vi "PH_Tektronix_7000.get Acquisition Configuration.vi"(0 "i ref in":refnum<vi>, 5 "error IO":errorcluster) -> (14 "i ref out":refnum<vi>, 19 "error out":errorcluster)   [LabVIEW 2014, in "PH_Tektronix_7000.lvlib"]
doc: "If the connection is established, the acquisition configuration is queried from the hardware and written to own attributes as well as the errors."
uses:
  PH_Tektronix_7000.lvlib
  PH_Tektronix_7000.Acquisition Config.ctl
  instr.lib/Tektronix7000Series/Tektronix 7000 Series - Driver np.lvlib
panel:
  in  "Acquisition Configuration":T1={"Record Length"=10000, "Timebase [s/div]"=4.0, "Position [%]"=0.0, "Acquisition Type"=0, "Average Waveforms"=10, "Envelope Waveforms"=10, "WfmDB Samples"=16000, "Continuous?"=FALSE, "Delay [s]"=0.0, "Run?"=FALSE} {"Delay [s]" format="%#_12p"; "Acquisition Type" items=["Sample", "Peak Detect", "Hi Res", "Average", "Envelope", "WfmDB"]; "Timebase [s/div]" format="%#_12g"}
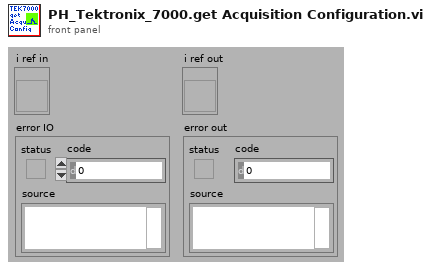
[diagram p1: front panel]
types:
  T1 = typedef "PH_Tektronix_7000.lvlib/PH_Tektronix_7000.Acquisition Config.ctl" = cluster{"Record Length":u32, "Timebase [s/div]":dbl, "Position [%]":dbl, "Acquisition Type":u16, "Average Waveforms":i32, "Envelope Waveforms":i32, "WfmDB Samples":i32, "Continuous?":bool, "Delay [s]":dbl, "Run?":bool}
  T2 = typedef "PH_Tektronix_7000.lvlib/PH_Tektronix_7000.i attribute.ctl" = cluster{"VISA Resource Name":refnum<visa-resource-name>, "IDN":cluster{"Instrument Driver":string, "Instrument Firmware":string, "Model":string, "Serial Number":string}, "Selftest":cluster{"Result":i32, "Message":string}, "Trigger Configuration":T3, "Acquisition Configuration":T1, "GUI Refs":T4, "State":T5, "Error Message":string, "Allow Prdc Loop?":bool, "Channel 1":T6, "Channel 2":T6, "Channel 3":T6, "Channel 4":T6, "Data CH 1":waveform(dbl), "Data CH 2":waveform(dbl), "Data CH 3":waveform(dbl), "Data CH 4":waveform(dbl), "Allow config?":bool, "Name Channel 1":string, "Name Channel 2":string, "Name Channel 3":string, "Name Channel 4":string, "Fetch Data before sending to PSDB?":bool, "Constructor passed?":bool, "Data taken at":timestamp, "Plot Colors":u32[], "Default VISA Resource":string}
  T3 = typedef "PH_Tektronix_7000.lvlib/PH_Tektronix_7000.Trigger Config.ctl" = cluster{"Source":u16, "Level [V]":dbl, "Slope":u16, "Coupling":u16, "Trigger Mode":u16}
  T4 = typedef "PH_Tektronix_7000.lvlib/PH_Tektronix_7000.GUI Refs.ctl" = cluster{"Graph":refnum<vi>, "State":refnum<vi>, "Delete":refnum<vi>, "VISA Resource":refnum<vi>, "Allow Configure":refnum<vi>, "Fetch Data":refnum<vi>, "Fetch before sending Data to PSDB":refnum<vi>, "Name Channel 1":refnum<vi>, "Name Channel 2":refnum<vi>, "Name Channel 3":refnum<vi>, "Name Channel 4":refnum<vi>, "Prdc Intervall [ms]":refnum<vi>, "Data taken":refnum<vi>, "Model":refnum<vi>, "Serial Number":refnum<vi>, "Firmware":refnum<vi>, "Driver":refnum<vi>, "Acquisition":refnum<vi>, "Trigger":refnum<vi>, "Cursor: D Time [s]":refnum<vi>, "Cursor: D Signal [V]":refnum<vi>, "Channel 1":refnum<vi>, "Channel 2":refnum<vi>, "Channel 3":refnum<vi>, "Channel 4":refnum<vi>}
  T5 = typedef "PH_StatusHandler.lvlib/PH_StatusHandler.Status.ctl" = i16
  T6 = typedef "PH_Tektronix_7000.lvlib/PH_Tektronix_7000.Channel Config.ctl" = cluster{"Enable Channel":bool, "Bandwidth":u16, "Input Impedance":u16, "Vertical Coupling":u16, "Probe Attenuation":dbl, "Range [V/div]":dbl, "Position [div]":dbl, "Bandwidth raw":string}
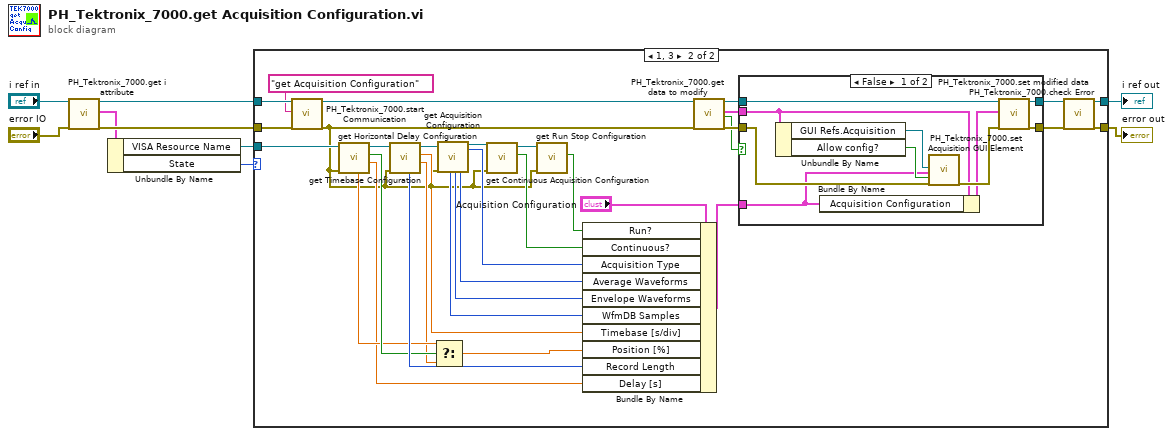
[diagram p0: block diagram]
diagram:
  n1 = call "PH_Tektronix_7000.get i attribute.vi"("i ref in"="i ref in", "error in (no error)"="error IO") -> ("i ref out"=w2:refnum<vi>, "i attribute"=w3:T2, "error out"=w5:errorcluster)  [unwired: 15 in]
  n2 = Unbundle By Name(w3) -> ("VISA Resource Name"=w4:refnum<visa-resource-name>, "State"=w1:T5)
  n3 = case shown="1, 3" w1 {
    tunnel: w2 -> [w11 w42]
    tunnel: w4 -> [_ w37]
    tunnel: [w10 w43] -> w8
    tunnel: w5 -> [w10 w44]
    tunnel: [w11 w41] -> w9
    frame Default {
    }
    frame 1, 3 {
      n4 = call "PH_Tektronix_7000.start Communication.vi"("i ref in"=w42, "Action"="get Acquisition Configuration", "error in"=w44) -> ("i ref out"=w35:refnum<vi>, "error out"=w12:errorcluster)  [unwired: 15 in]
      n5 = call "get Horizontal Delay Configuration.vi"("error in (no error)"=w12, "VISA resource name"=w37) -> ("Delay [s]"=w15:dbl, "Delay activated?"=w19:bool, "VISA resource name out"=w20:refnum<visa-resource-name>, "Position [%]"=w18:dbl)  [unwired: 5 in, 1 out]
      n6 = call "get Timebase Configuration.vi"("error in (no error)"=w12, "VISA resource name"=w20) -> ("Position [%]"=w17:dbl, "Timebase [s]"=w22:dbl, "VISA resource name out"=w39:refnum<visa-resource-name>, "Record Length"=w23:u32)  [unwired: 5 in, 1 out]
      n7 = Select(t=w18, s=w19, f=w17) -> (s? t:f=w16:dbl)
      n8 = call "get Acquisition Configuration.vi"("VISA resource name"=w39, "error in (no error)"=w12) -> ("WfmDB Samples"=w24:i32, "Envelope Waveforms"=w25:i32, "Average Waveforms"=w26:i32, "VISA resource name out"=w38:refnum<visa-resource-name>, "Acquisition Type"=w27:u16)  [unwired: 9 in, 4 out]
      n9 = call "get Continuous Acquisition Configuration.vi"("VISA resource name"=w38, "error in (no error)"=w12) -> ("VISA resource name out"=w14:refnum<visa-resource-name>, "Continuous Acquisition Mode"=w28:bool)  [unwired: 5 in, 2 out]
      n10 = call "get Run Stop Configuration.vi"("VISA resource name"=w14, "error in (no error)"=w12) -> ("Continuous Acquisition Mode"=w13:bool)  [unwired: 5 in, 3 out]
      n11 = Bundle By Name(cluster="Acquisition Configuration", "Run?"=w13, "Continuous?"=w28, "Acquisition Type"=w27, "Average Waveforms"=w26, "Envelope Waveforms"=w25, "WfmDB Samples"=w24, "Timebase [s/div]"=w22, "Position [%]"=w16, "Record Length"=w23, "Delay [s]"=w15) -> (w21:T1)
      n12 = call "PH_Tektronix_7000.get data to modify.vi"("i ref in"=w35, "error in (no error)"=w12) -> ("i ref out"=w32:refnum<vi>, "i attribute"=w30:T2, "timed out"=w33:bool, "error out"=w36:errorcluster)  [unwired: 14 in]
      n13 = case shown="False" w33 {
        tunnel: w36 -> [w54 w56]
        tunnel: [w53 w56] -> w34
        tunnel: w32 -> [w51 w55]
        tunnel: [w50 w55] -> w31
        tunnel: w30 -> [w48 _]
        tunnel: w21 -> [w46 _]
        frame False {
          n14 = Unbundle By Name(w48) -> ("GUI Refs.Acquisition"=w45:refnum<vi>, "Allow config?"=w47:bool)
          n15 = Bundle By Name(cluster=w48, "Acquisition Configuration"=w46) -> (w49:T2)
          n16 = call "PH_Tektronix_7000.set Acquisition GUI Element.vi"("Ref Acqu Config"=w45, "Acqu Config"=w46, "enabled?"=w47, "error in"=w54) -> ("error out"=w52:errorcluster)  [unwired: 15 in]
          n17 = call "PH_Tektronix_7000.set modified data.vi"("i ref in"=w51, "i attribute"=w49, "error in (no error)"=w52) -> ("i ref out"=w50:refnum<vi>, "error out"=w53:errorcluster)  [unwired: 15 in]
        }
        frame True {
        }
      }
      n18 = call "PH_Tektronix_7000.check Error.vi"("i ref in"=w31, "error in"=w34) -> ("i ref out"=w41:refnum<vi>, "error out"=w43:errorcluster)  [unwired: 16 in]
    }
  }
  "i ref out" <- w9
  "error out" <- w8
